vi "niScope Initialize Virtual Channels.vi"(8 "error in":errorcluster, 10 "Reset card (False)":bool, 11 "niScope in":T1={"channel cfg"=[], "sessions"=[], "multi cards"=FALSE, "channels"=0, "type"=enum."n/a", "memory [B/chn]"=0, "ext. clock [Hz]"=0.0, "samples count"=0, "use streaming"=FALSE, "proc setup"={"packet size [smpl]"=0, "current timeout [s]"=0.0, "blk2blk timeout [s]"=0.0, "event time"=timestamp(0 s since 1904-01-01), "temp sampl T [s]"=0.0, "data queue"=refnum, "stop notifier"=refnum, "proc ref"=refnum}, "sample width [B]"=0, "ranges [V]"=[], "trigger setup"={"coupling"=1, "level [V]"=0.0, "slope"=0, "mode"=enum."Immediate"}, "fs [Hz]"=0.0, "bitres [bit]"=0} {"trigger setup"."level [V]" format="%.2f"; "trigger setup"."coupling" items=["AC"=0, "DC"=1, "HF Reject"=3, "LF Reject"=4, "AC Plus HF Reject"=1001]; "channel cfg"."Range [Vpk]" min=0.0; "channel cfg"."Channel" min=0}) -> (0 "error out":errorcluster, 1 "idn strings":string[](array[string]), 2 "combined idn string":string, 3 "niScope out":T1={"channel cfg"=[], "sessions"=[], "multi cards"=FALSE, "channels"=0, "type"=enum."n/a", "memory [B/chn]"=0, "ext. clock [Hz]"=0.0, "samples count"=0, "use streaming"=FALSE, "proc setup"={"packet size [smpl]"=0, "current timeout [s]"=0.0, "blk2blk timeout [s]"=0.0, "event time"=timestamp(0 s since 1904-01-01), "temp sampl T [s]"=0.0, "data queue"=refnum, "stop notifier"=refnum, "proc ref"=refnum}, "sample width [B]"=0, "ranges [V]"=[], "trigger setup"={"coupling"=1, "level [V]"=0.0, "slope"=0, "mode"=enum."Immediate"}, "fs [Hz]"=0.0, "bitres [bit]"=0} {"trigger setup"."level [V]" format="%.2f"; "trigger setup"."coupling" items=["AC"=0, "DC"=1, "HF Reject"=3, "LF Reject"=4, "AC Plus HF Reject"=1001]; "channel cfg"."Range [Vpk]" min=0.0; "channel cfg"."Channel" min=0})   [LabVIEW 2018, in "niScope Virtual Digitizer.lvlib"]
doc: "Identification and initialization of the cards used in the virtual channels list. Only supported models will be allowed and all cards in the virtual channels must be the same. This VI must be called before using any other top level function dealing with the virtual channels."
uses:
  niScope Virtual Digitizer.lvlib
  niScope Session.ctl
  niScope Virtual Channel Config.ctl
  niScope Virtual Channel Mode.ctl
  niScope Virtual Channel Input Z.ctl
  niScope Virtual Channel Coupling.ctl
  niScope Type.ctl
  niScope Digitizing Process Options.ctl
  niScope Data Packet.ctl
  niScope Trigger Setup.ctl
  <instrlib>/niScope/Controls/niScope trigger coupling.ctl
  <instrlib>/niScope/Controls/niScope trigger slope.ctl
  <vilib>/Utility/error.llb/Error Cluster From Error Code.vi
  <vilib>/ErrorRing/Error Ring.xnode
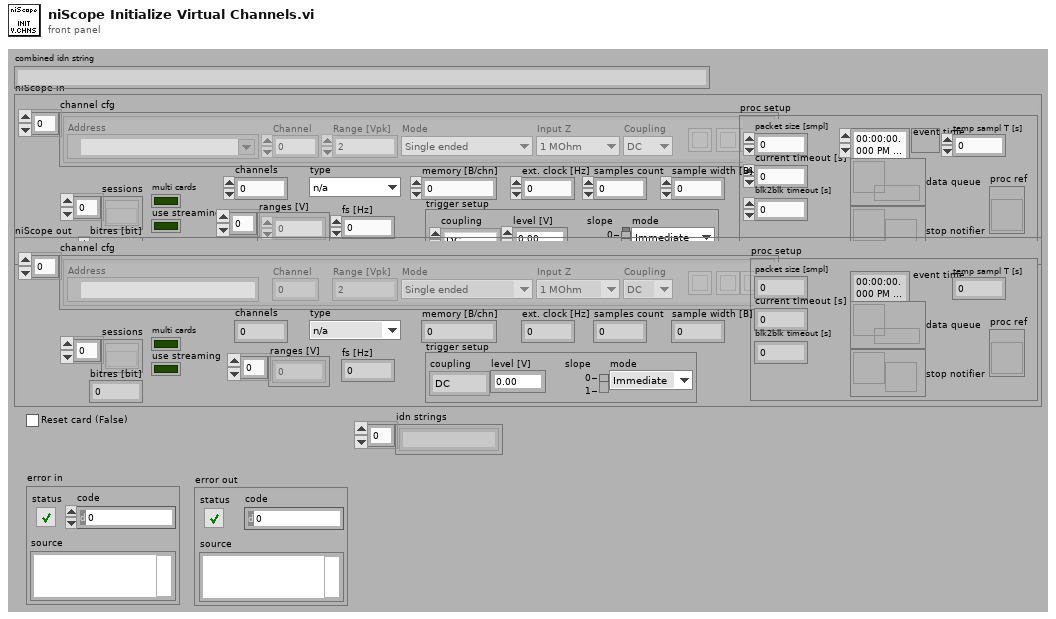
[diagram p1: front panel]
types:
  T1 = typedef "niScope Virtual Digitizer.lvlib/niScope Session.ctl" = cluster{"channel cfg":T2[], "sessions":refnum<k20>[], "multi cards":bool, "channels":i32, "type":T6, "memory [B/chn]":i32, "ext. clock [Hz]":dbl, "samples count":i64, "use streaming":bool, "proc setup":T7, "sample width [B]":i32, "ranges [V]":dbl[], "trigger setup":T8, "fs [Hz]":dbl, "bitres [bit]":i32}
  T2 = typedef "niScope Virtual Digitizer.lvlib/niScope Virtual Channel Config.ctl" = cluster{"Address":refnum<k15>, "Channel":i32, "Mode":T3, "Input Z":T4, "Coupling":T5, "Range [Vpk]":dbl, "btn clr":bool, "btn up":bool, "btn down":bool}
  T3 = typedef "niScope Virtual Digitizer.lvlib/niScope Virtual Channel Mode.ctl" = enum16{"Single ended", "Unbal. differential", "Differential"}
  T4 = typedef "niScope Virtual Digitizer.lvlib/niScope Virtual Channel Input Z.ctl" = enum16{"1 MOhm", "50 Ohm"}
  T5 = typedef "niScope Virtual Digitizer.lvlib/niScope Virtual Channel Coupling.ctl" = enum16{"AC", "DC", "GND"}
  T6 = typedef "niScope Virtual Digitizer.lvlib/niScope Type.ctl" = enum16{"n/a", "5922"}
  T7 = typedef "niScope Virtual Digitizer.lvlib/niScope Digitizing Process Options.ctl" = cluster{"packet size [smpl]":i64, "current timeout [s]":dbl, "blk2blk timeout [s]":dbl, "event time":timestamp, "temp sampl T [s]":dbl, "data queue":refnum<queue>, "stop notifier":refnum<notifier>, "proc ref":refnum<vi>}
  T8 = typedef "niScope Virtual Digitizer.lvlib/niScope Trigger Setup.ctl" = cluster{"coupling":T9, "level [V]":dbl, "slope":T10, "mode":enum16{"Immediate", "External", "Level"}}
  T9 = typedef "niScope trigger coupling.ctl" = u16
  T10 = typedef "niScope trigger slope.ctl" = i32
  T11 = typedef "niScope Virtual Digitizer.lvlib/niScope Physical Cards.ctl" = cluster{"chn lst":i32[], "addr":refnum<k15>, "chn pos":i32[]}
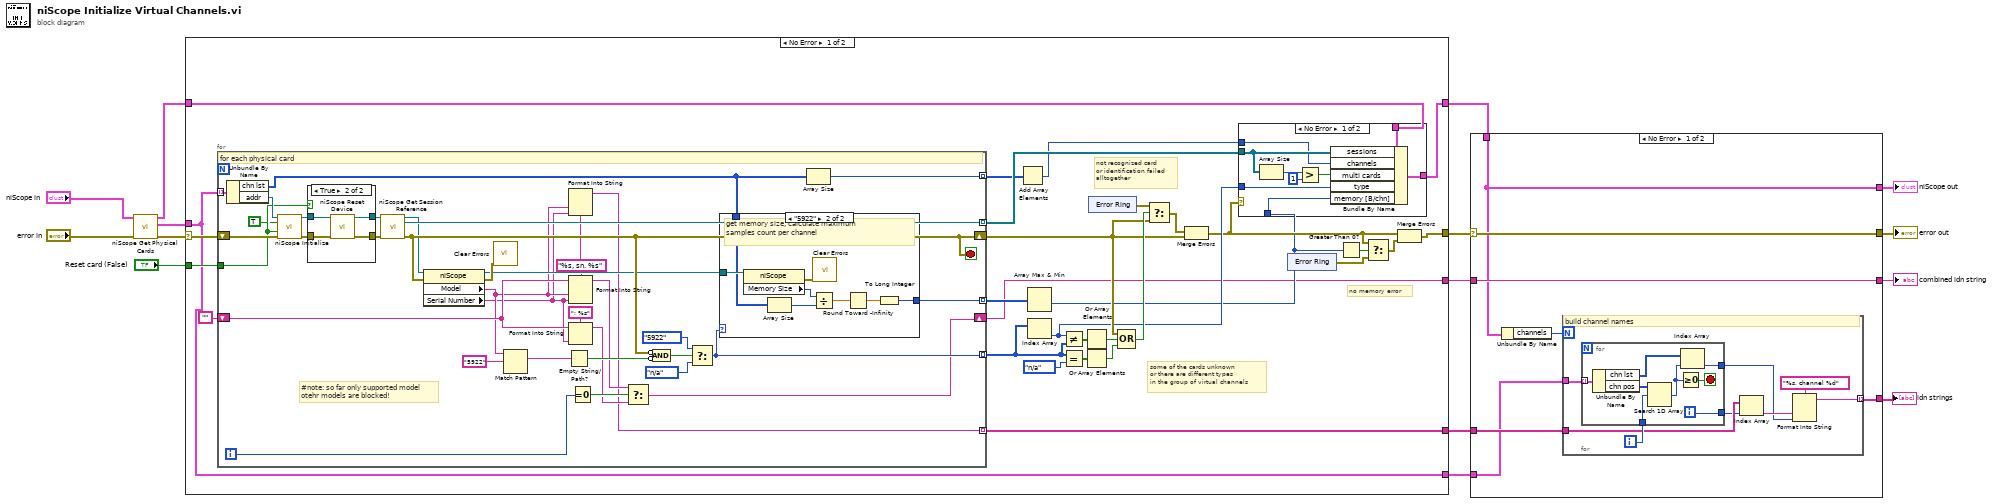
[diagram p0: block diagram]
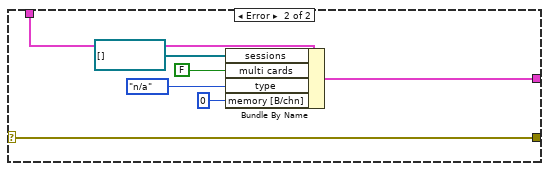
[diagram p2: hidden frame]
diagram:
  n1 = call "niScope Get Physical Cards.vi"("error in"="error in", "niScope in"="niScope in") -> ("error out"=w11:errorcluster, "card list"=w15:T11[], "niScope out"=w10:T1)  [unwired: 7 in]
  n2 = case shown="No Error" w11 {
    selector: w11 -> [w43 w114]
    tunnel: w15 -> [w16 _]
    tunnel: "Reset card (False)" -> [w44 _]
    tunnel: w10 -> [w31 w115]
    tunnel: [w27 w114] -> w9
    tunnel: [w28 w115] -> w8
    tunnel: [w18 _] -> w5
    tunnel: [w17 _] -> w3
    tunnel: [w16 _] -> w1
    frame No Error {
      # "no memory error"
      # "not recognized card\nor identification failed\nalltogether"
      # "some of the cards unknown\nor there are different types\nin the group of virtual channels"
      n3 = for {
        tunnel: w44 -> [w91]
        shift-right: [w70] -> w18
        shift-left: "" -> [w71]
        shift-right: [w82] -> w33
        shift-left: w43 -> [w99]
        tunnel: [w90] -> w30 mode=indexing
        tunnel: w16 -> [w97] mode=indexing
        tunnel: [w78] -> w39 mode=indexing
        tunnel: [w79] -> w24 mode=indexing
        tunnel: [w76] -> w20 mode=indexing
        tunnel: [w65] -> w17 mode=indexing
        i -> [w74]
        stop <- w82 stop-if-true
        w68 = "%s, sn. %s" ("format string")
        # "#note: so far only supported model\notehr models are blocked!"
        # "for each physical card"
        n4 = Unbundle By Name(w97) -> ("chn lst"=w77:i32[], "addr"=w96:refnum<k15>)
        n5 = call <instrlib>:"niScope Initialize.vi"("resource name"=w96, "id query"=TRUE, "reset device"=w91, "error in"=w99) -> ("instrument handle"=w94:refnum<k15>, "error out"=w95:errorcluster)  [unwired: 10 in]
        n6 = case shown="True" w91 {
          tunnel: w95 -> [w109 w113]
          tunnel: w94 -> [w108 w110]
          tunnel: [w109 w112] -> w93
          tunnel: [w108 w111] -> w92
          frame False {
          }
          frame True {
            n7 = call <instrlib>:"niScope Reset Device.vi"("instrument handle"=w110, "error in"=w113) -> ("instrument handle out"=w111:refnum<k15>, "error out"=w112:errorcluster)  [unwired: 12 in]
          }
        }
        n8 = call <instrlib>:"niScope Get Session Reference.vi"("instrument handle"=w92, "error in"=w93) -> ("instrument handle out"=w81:refnum<k15>, "session reference"=w90:refnum<k20>, "error out"=w82:errorcluster)  [unwired: 11 in]
        n9 = property class="niScope"(reference=w81, error in=w82) -> (reference out=w80:refnum<k15>, error out=w98:errorcluster, "Model"=w67:string, "Serial Number"=w66:string)
        n10 = call <vilib>:"Clear Errors.vi"("error in (no error)"=w98) -> ()  [unwired: 5 in, 2 out]
        n11 = Match Pattern(string=w67, regular expression="5922") -> (match substring=w87:string)  [unwired: 1 in, 3 out]
        n12 = Empty String/Path?(string/path=w87) -> (empty?=w86:bool)
        n13 = Format Into String(format string=w68, w67, w66) -> (resulting string=w65:string)  [unwired: 2 in, 1 out]
        n14 = Format Into String(format string="; %s", initial string=w71, w66) -> (resulting string=w72:string)  [unwired: 1 in, 1 out]
        n15 = Format Into String(format string=w68, initial string=w71, w67, w66) -> (resulting string=w69:string)  [unwired: 1 in, 1 out]
        n16 = Equal To 0?(x=w74) -> (x = 0?=w73:bool)
        n17 = Select(t=w69, s=w73, f=w72) -> (s? t:f=w70:string)
        n18 = Compound Arithmetic op=AND(invert w82, invert w86) -> (w85:bool)
        n19 = Select(t=niScope_Type."5922" ("type"), s=w85, f=niScope_Type."n/a" ("type")) -> (s? t:f=w78:T6)
        n20 = case shown="\"5922\"" w78 {
          tunnel: w80 -> [_ w106]
          tunnel: w77 -> [_ w104]
          tunnel: [_ w103] -> w79
          frame Default {
          }
          frame "5922" {
            # "get memory size, calculate maximum \nsamples count per channel"
            n21 = property class="niScope"(reference=w106) -> (error out=w107:errorcluster, "Memory Size"=w105:i32)  [unwired: 1 in, 1 out]
            n22 = Array Size(array=w104) -> (size(s)=w102:i32)
            n23 = Divide(x=w105, y=w102) -> (x/y=w101:dbl)
            n24 = call <vilib>:"Clear Errors.vi"("error in (no error)"=w107) -> ()  [unwired: 5 in, 2 out]
            n25 = Round Toward -Infinity(1:w101) -> (0:w100:dbl)
            n26 = To Long Integer(number=w100) -> (32bit integer=w103:i32)
          }
        }
        n27 = Array Size(array=w77) -> (size(s)=w76:i32)
      }
      n28 = Add Array Elements(numeric array=w20) -> (sum=w19:i32)
      n29 = Array Max & Min(array=w24) -> (min value=w21:i32)  [unwired: 3 out]
      n30 = Index Array(array=w39) -> (element=w29:T6)  [unwired: 1 in]
      n31 = Not Equal?(x=w29, y=w39) -> (x != y?=w38:bool[])
      n32 = Equal?(x=w39, y=niScope_Type."n/a" ("type")) -> (x = y?=w40:bool[])
      n33 = Or Array Elements(Boolean array=w38) -> (logical OR=w37:bool)
      n34 = Or Array Elements(Boolean array=w40) -> (logical OR=w36:bool)
      n35 = xnode "Error Ring"() -> ("error out"=w32:errorcluster)
      n36 = Compound Arithmetic op=OR(w33, w37, w36) -> (w35:bool)
      n37 = Select(t=w32, s=w35, f=w33) -> (s? t:f=w34:errorcluster)
      n38 = Merge Errors(w34, w33) -> (w25:errorcluster)
      n39 = case shown="No Error" w25 {
        tunnel: w31 -> [w58 w59]
        tunnel: w30 -> [w57 _]
        tunnel: w29 -> [w53 _]
        tunnel: [w52 w59] -> w28
        tunnel: w21 -> [w51 _]
        tunnel: w19 -> [w50 _]
        frame No Error {
          n40 = Array Size(array=w57) -> (size(s)=w54:i32)
          n41 = Greater?(x=w54, y=1) -> (0:w55:bool)
          n42 = Bundle By Name(cluster=w58, "sessions"=w57, "channels"=w50, "multi cards"=w55, "type"=w53, "memory [B/chn]"=w51) -> (w52:T1)
        }
        frame Error {
        }
      }
      n43 = xnode "Error Ring"() -> ("error out"=w22:errorcluster)
      n44 = Greater Than 0?(x=w21) -> (x > 0?=w23:bool)
      n45 = Select(t=w25, s=w23, f=w22) -> (s? t:f=w26:errorcluster)
      n46 = Merge Errors(w25, w26) -> (w27:errorcluster)
    }
    frame Error {
    }
  }
  n47 = case shown="No Error" w9 {
    selector: w9 -> [w122 w140]
    tunnel: w8 -> [w117 w145]
    tunnel: [w117 w141] -> w6
    tunnel: [w122 w140] -> w7
    tunnel: w5 -> [w121 _]
    tunnel: [w121 _] -> w4
    tunnel: [w119 _] -> w2
    tunnel: w3 -> [w120 _]
    tunnel: w1 -> [w118 _]
    frame No Error {
      n48 = Unbundle By Name(w117) -> ("channels"=w116:i32)
      n49 = for {
        N: w116 -> [_]
        tunnel: w118 -> [w130]
        tunnel: w120 -> [w127]
        tunnel: [w123] -> w119 mode=indexing
        i -> [w129]
        # "build channel names"
        n50 = for {
          tunnel: w130 -> [w138] mode=indexing
          tunnel: w129 -> [w136]
          tunnel: [w134] -> w126
          tunnel: [w131] -> w124
          i -> [w134]
          stop <- w135 stop-if-true
          n51 = Unbundle By Name(w138) -> ("chn lst"=w132:i32[], "chn pos"=w137:i32[])
          n52 = Search 1D Array(1D array=w137, element=w136) -> (index of element=w133:i32)  [unwired: 1 in]
          n53 = Greater Or Equal To 0?(x=w133) -> (x >= 0?=w135:bool)
          n54 = Index Array(array=w132, index=w133) -> (element=w131:i32)
        }
        n55 = Index Array(array=w127, index=w126) -> (element=w125:string)
        n56 = Format Into String(format string="%s, channel %d", w125, w124) -> (resulting string=w123:string)  [unwired: 2 in, 1 out]
      }
    }
    frame Error {
      n57 = Bundle By Name(cluster=w145, "sessions"=refnum<k20>[] [], "multi cards"=FALSE, "type"=niScope_Type."n/a", "memory [B/chn]"=0 ("memory [smpl/chn]")) -> (w141:T1)
    }
  }
  "niScope out" <- w6
  "error out" <- w7
  "combined idn string" <- w4
  "idn strings" <- w2
